vi "Enable OutPut State.vi"(8 "error in":errorcluster, 10 "State":bool, 11 "VISA resource name":refnum<visa-resource-name>) -> (0 "error out":errorcluster, 3 "VISA resource name out":refnum<visa-resource-name>)   [LabVIEW 2018, in "IT-M3100.lvlib"]
doc: "This command sets the output state of the power supply.\n<b>State</b>\n0:Close the State\n1:Open the state"
uses:
  IT-M3100.lvlib
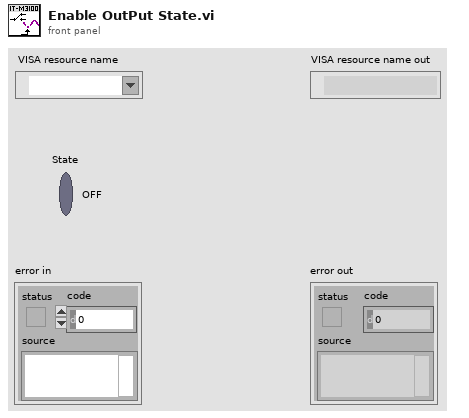
[diagram p1: front panel]
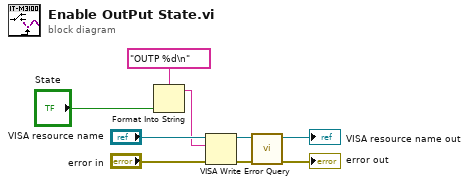
[diagram p0: block diagram]
diagram:
  n1 = Format Into String(format string="OUTP %d\n", "State") -> (resulting string=w1:string)  [unwired: 2 in, 1 out]
  n2 = VISA Write(VISA resource name="VISA resource name", write buffer=w1, error in (no error)="error in") -> (VISA resource name out=w6:refnum<visa-resource-name>, error out=w7:errorcluster)  [unwired: 1 out]
  n3 = call "Error Query.vi"("error in"=w7, "VISA resource name"=w6) -> ("error out"=→"error out":errorcluster, "VISA resource name out"=→"VISA resource name out":refnum<visa-resource-name>)  [unwired: 6 in, 2 out]
